vi "Day 01.vi"() -> ()   [LabVIEW 2021]
uses:
  <vilib>/addons/_JKI Toolkits/Caraya/classes/Assert/Assert Equal Value_Variant.vi
  <vilib>/addons/_JKI Toolkits/Caraya/classes/Assert/Assert.lvclass
  <vilib>/addons/_JKI Toolkits/Caraya/classes/Test/Test.lvclass
panel:
  out "Solution Part 2":i16
  in  "Part":enum16{"Part 1", "Part 2"}(ring)
  out "Solution Part 1":i16
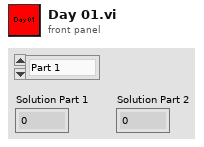
[diagram p1: front panel]
types:
  T1 = cluster{"Result Part1":i32, "Result Part2":i32, "Input":string}
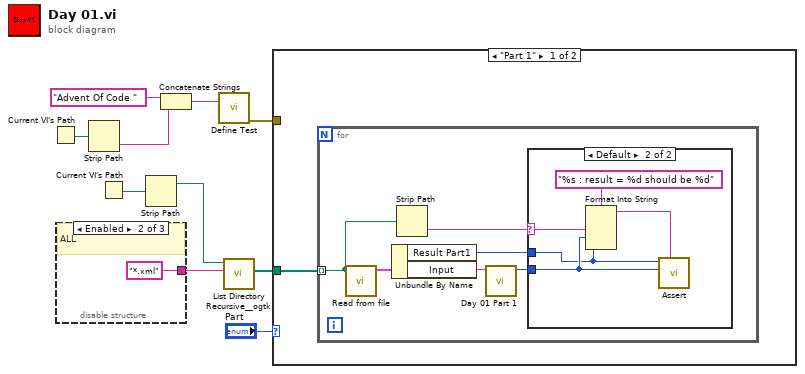
[diagram p0: block diagram]
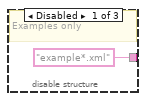
[diagram p2: hidden frame]
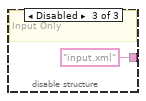
[diagram p3: hidden frame]
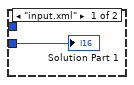
[diagram p4: hidden frame]
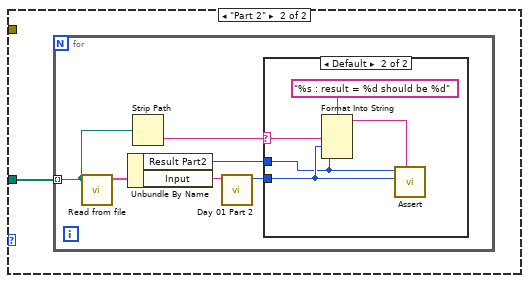
[diagram p5: hidden frame]
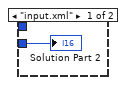
[diagram p6: hidden frame]
diagram:
  n1 = Current VI's Path() -> (path=w3:path)
  n2 = disable-structure shown="Enabled" {
    disable-tunnel: ["example*.xml" ("pattern") "*.xml" ("pattern") "input.xml" ("pattern")] -> w8
    frame Disabled {
      # "Examples only"
    }
    frame Enabled {
      # "ALL"
    }
    frame Disabled {
      # "Input Only"
    }
  }
  n3 = Strip Path(path=w3) -> (name=w1:string)  [unwired: 1 out]
  n4 = Current VI's Path() -> (path=w10:path)
  n5 = Strip Path(path=w10) -> (stripped path=w9:path)  [unwired: 1 out]
  n6 = Concatenate Strings("Advent Of Code " ("Label (VI Title)"), w1) -> (w2:string)
  n7 = call <vilib>:"Define Test.vi"("Label (VI Title)"=w2) -> ("error out"=w5:errorcluster)  [unwired: 10 in]
  n8 = call <userlib>:"List Directory Recursive__ogtk.vi"("pattern"=w8, "Path"=w9) -> ("file paths"=w6:path[])  [unwired: 6 in, 3 out]
  n9 = case shown="\"Part 1\"" "Part" {
    tunnel: w6 -> [w14 w27]
    tunnel: w5 -> [_ _]
    frame "Part 1" {
      n10 = for {
        tunnel: w14 -> [w17] mode=indexing
        n11 = call "Read from file.vi"("File Path"=w17) -> ("Data"=w19:T1)  [unwired: 10 in]
        n12 = Unbundle By Name(w19) -> ("Result Part1"=w18:i32, "Input"=w20:string)
        n13 = Strip Path(path=w17) -> (name=w16:string)  [unwired: 1 out]
        n14 = call "Day 01 Part 1.vi"("Input"=w20) -> ("Output"=w15:i16)  [unwired: 10 in]
        n15 = case shown="Default" w16 {
          selector: w16 -> [_ w26]
          tunnel: w18 -> [_ w22]
          tunnel: w15 -> [w21 w23]
          frame "input.xml" {
            "Solution Part 1" <- w21
          }
          frame Default {
            n16 = Format Into String(format string="%s : result = %d should be %d", w26, w23, w22) -> (resulting string=w25:string)  [unwired: 2 in, 1 out]
            n17 = call-poly <vilib>:"Assert.vi"("Label"=w25, "Y"=w23, "X"=w22) -> ()  [unwired: 8 in, 1 out]
          }
        }
      }
    }
    frame "Part 2" {
      n18 = for {
        tunnel: w27 -> [w30] mode=indexing
        n19 = call "Read from file.vi"("File Path"=w30) -> ("Data"=w32:T1)  [unwired: 10 in]
        n20 = Unbundle By Name(w32) -> ("Result Part2"=w31:i32, "Input"=w33:string)
        n21 = Strip Path(path=w30) -> (name=w29:string)  [unwired: 1 out]
        n22 = call "Day 01 Part 2.vi"("Input"=w33) -> ("Output"=w28:i16)  [unwired: 10 in]
        n23 = case shown="Default" w29 {
          selector: w29 -> [_ w39]
          tunnel: w31 -> [_ w35]
          tunnel: w28 -> [w34 w36]
          frame "input.xml" {
            "Solution Part 2" <- w34
          }
          frame Default {
            n24 = Format Into String(format string="%s : result = %d should be %d", w39, w36, w35) -> (resulting string=w38:string)  [unwired: 2 in, 1 out]
            n25 = call-poly <vilib>:"Assert.vi"("Label"=w38, "Y"=w36, "X"=w35) -> ()  [unwired: 8 in, 1 out]
          }
        }
      }
    }
  }
